vi "tmp_toml_type_cast.vi"(7 "action":enum8{"get", "set"}(ring), 8 "error in (no error)":errorcluster, 10 "item":T1, 11 "text in":string) -> (0 "error out":errorcluster, 1 "exists?":bool, 2 "value":variant, 3 "text out":string)   [LabVIEW 2017]
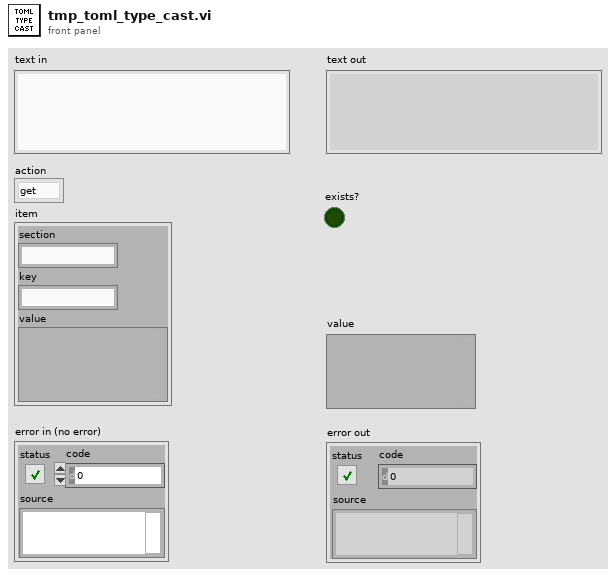
[diagram p1: front panel]
types:
  T1 = cluster{"section":string, "key":string, "value":variant}
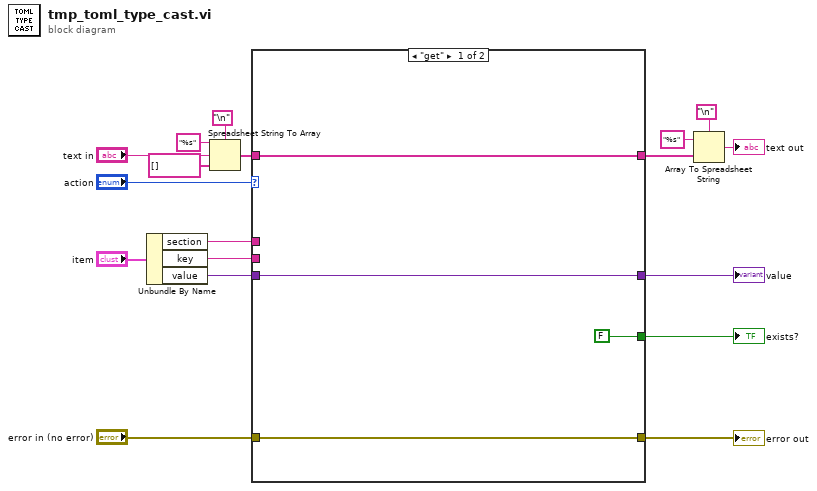
[diagram p0: block diagram]
diagram:
  n1 = Unbundle By Name("item") -> ("section"=w14:string, "key"=w13:string, "value"=w12:variant)
  n2 = Spreadsheet String To Array(delimiter (Tab)="\n", format string="%s", spreadsheet string="text in", array type (2D Dbl)=string[] []) -> (array=w6:string[])
  n3 = case shown="\"get\"" "action" {
    tunnel: [w22 w25] -> w5
    tunnel: w6 -> [w22 w25]
    tunnel: [w21 w24] -> w16
    tunnel: "error in (no error)" -> [w21 w24]
    tunnel: w14 -> [_ _]
    tunnel: w13 -> [_ _]
    tunnel: w12 -> [w20 w23]
    tunnel: [w20 w23] -> w11
    tunnel: [FALSE ("exists?") _] -> w1
    frame "get" {
    }
    frame "set" {
    }
  }
  "error out" <- w16
  "value" <- w11
  "exists?" <- w1
  n4 = Array To Spreadsheet String(delimiter (Tab)="\n", array=w5, 3:"%s" ("format string")) -> (spreadsheet string=→"text out":string)
